vi "send_all.vi"(2 "current time":timestamp, 3 "names":string[](array[string]), 4 "error IO":errorcluster, 5 "Boolean":bool, 6 "Time Stamp":timestamp, 7 "directory dup":path) -> (0 "error out":errorcluster, 1 "last ses time":timestamp)   [LabVIEW 2010]
uses:
  Global 2.vi
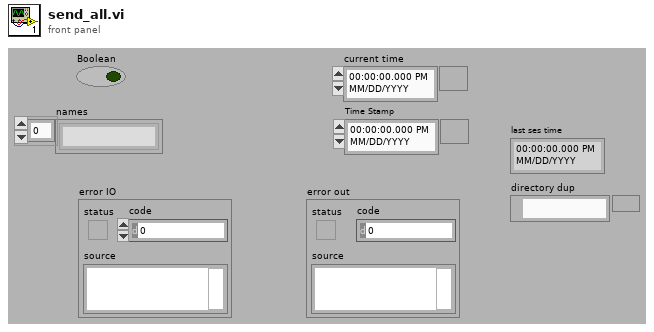
[diagram p1: front panel]
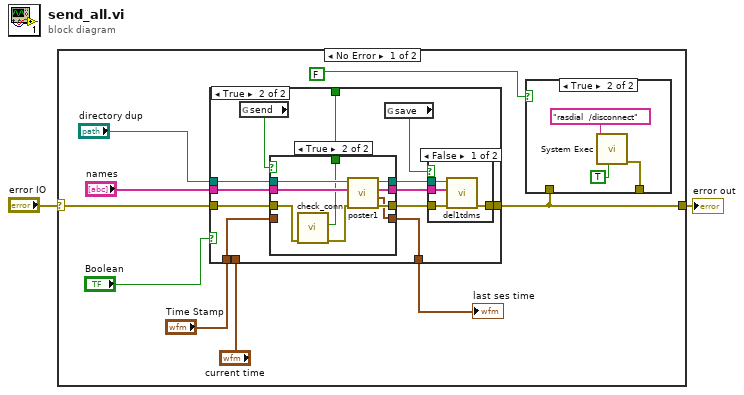
[diagram p0: block diagram]
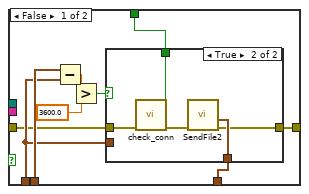
[diagram p3: hidden frame]
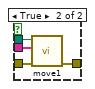
[diagram p6: hidden frame]
diagram:
  n1 = case shown="No Error" "error IO" {
    selector: "error IO" -> [w5 w67]
    tunnel: [w4 w67] -> w2
    frame No Error {
      n2 = case shown="True" "Boolean" {
        tunnel: "directory dup" -> [_ w44]
        tunnel: "names" -> [_ w40]
        tunnel: w5 -> [w17 w34]
        tunnel: [w20 w37] -> w9
        tunnel: "Time Stamp" -> [w19 w36]
        tunnel: "current time" -> [w24 _]
        tunnel: [w18 w35] -> w4
        tunnel: [w16 w33] -> _
        frame False {
          n3 = Subtract(x=w24, y=w19) -> (x-y=w23:dbl)
          n4 = Greater?(x=w23, y=3600.0) -> (0:w21:bool)
          n5 = case shown="True" w21 {
            selector: w21 -> [w25 _]
            tunnel: [w27 w32] -> w20
            tunnel: w19 -> [w27 _]
            tunnel: [w26 w31] -> w18
            tunnel: w17 -> [w26 w30]
            tunnel: [w25 w29] -> w16
            frame False {
            }
            frame True {
              n6 = call "check_conn.vi"("error in (no error)"=w30) -> ("error out"=w28:errorcluster, "modem used"=w29:bool)  [unwired: 5 in]
              n7 = call "SendFile2.vi"("error in"=w28) -> ("error out"=w31:errorcluster, "last ses time"=w32:timestamp)  [unwired: 5 in]
            }
          }
        }
        frame True {
          n8 = global read "Global 2.vi" "send"() -> (w38:bool)
          n9 = case shown="True" w38 {
            selector: w38 -> [w45 _]
            tunnel: w44 -> [w47 w58]
            tunnel: w40 -> [w49 w55]
            tunnel: [w47 w57] -> w43
            tunnel: [w49 w54] -> w42
            tunnel: [w48 w56] -> w41
            tunnel: w34 -> [w48 w52]
            tunnel: [w46 w53] -> w37
            tunnel: w36 -> [w46 _]
            tunnel: [w45 w50] -> w33
            frame False {
            }
            frame True {
              n10 = call "check_conn.vi"("error in (no error)"=w52) -> ("error out"=w51:errorcluster, "modem used"=w50:bool)  [unwired: 5 in]
              n11 = call "poster1.vi"("error in"=w51, "subarray"=w55, "dir path"=w58) -> ("error out"=w56:errorcluster, "last ses time"=w53:timestamp, "names"=w54:string[], "dir"=w57:path)  [unwired: 1 in]
            }
          }
          n12 = global read "Global 2.vi" "save"() -> (w39:bool)
          n13 = case shown="False" w39 {
            tunnel: w43 -> [w62 w63]
            tunnel: w42 -> [w59 w64]
            tunnel: w41 -> [w61 w66]
            tunnel: [w60 w65] -> w35
            frame False {
              n14 = call "del1tdms.vi"("error in (no error)"=w61, "names"=w59, "sent time file path"=w62) -> ("error out"=w60:errorcluster)  [unwired: 4 in]
            }
            frame True {
              n15 = call "move1.vi"("error in (no error)"=w66, "names"=w64, "dir path"=w63) -> ("error out"=w65:errorcluster)  [unwired: 4 in]
            }
          }
        }
      }
      "last ses time" <- w9
      n16 = case shown="True" FALSE ("run minimized? (F)") {
        tunnel: w4 -> [w12 _]
        tunnel: [w12 w13] -> _
        frame False {
        }
        frame True {
          n17 = call <vilib>:"System Exec.vi"("run minimized? (F)"=TRUE, "command line"="rasdial  /disconnect") -> ("error out"=w13:errorcluster)  [unwired: 6 in, 3 out]
        }
      }
    }
    frame Error {
    }
  }
  "error out" <- w2
